vi "Fetch Waveform Measurement.vi"(6 "Source 2 (21: None)":u16(ring)=21 items=["Channel 1", "Channel 2", "Channel 3", "Channel 4", "DIG 0", "DIG 1", "DIG 2", "DIG 3", "DIG 4", "DIG 5", "DIG 6", "DIG 7", "DIG 8", "DIG 9", "DIG 10", "DIG 11", "DIG 12", "DIG 13", "DIG 14", "DIG 15", "Math", "None"], 8 "error in (no error)":errorcluster, 9 "Measurement Function (7: Frequency)":u16(ring)=7 items=["Amplitude", "Voltage Average", "Base", "Counter", "Delay", "Duty Cycle", "Fall Time", "Frequency", "Voltage Max", "Voltage Min", "Overshoot", "Voltage Vpp", "Period", "Phase", "Preshoot", "Rise Time", "Voltage RMS", "Top", "Width Positive", "X at Max Y", "X at Min Y"], 10 "Source 1 (0: Channel 1)":u16(ring) items=["Channel 1", "Channel 2", "Channel 3", "Channel 4", "DIG 0", "DIG 1", "DIG 2", "DIG 3", "DIG 4", "DIG 5", "DIG 6", "DIG 7", "DIG 8", "DIG 9", "DIG 10", "DIG 11", "DIG 12", "DIG 13", "DIG 14", "DIG 15", "Math"], 11 "VISA resource name":refnum<visa-resource-name>) -> (0 "error out":errorcluster, 2 "Measured Value":dbl, 3 "VISA resource name out":refnum<visa-resource-name>)   [LabVIEW 2018, in "Agilent 6000 Series.lvlib"]
doc: "This VI obtains a waveform measurement and returns the measurement value. You specify a particular measurement type, such as rise time, frequency, and voltage peak-to-peak. The waveform on which the oscilloscope calculates the waveform measurement is from an acquisition that you previously initiated. \n\nUse the ag6000 Initiate Acquisition.vi to start an acquisition on the channels that you enable with the ag6000 Configure Channel.vi. The oscilloscope acquires waveforms for the enabled channels concurrently. You use the ag6000 Acquisition Status.vi to determine when the acquisition is complete. You call this VI separately for each waveform measurement you want to obtain on a specific channel.\n\nYou can call the ag6000 Read Waveform Measurement.vi instead of the ag6000 Initiate Acquisition.vi. The ag6000 Read Waveform Measurement.vi starts an acquisition on all enabled channels. It then waits for the acquisition to complete, obtains a waveform measurement on the channel you specify, and returns the measurement value. You call this VI separately for any other waveform measurement that you want to obtain on a specific channel.\n\nNotes:\n\n(1) You must configure the appropriate reference levels before you call this VI to take a rise time, fall time, width negative, width positive, duty cycle negative, or duty cycle positive measurement.\n\n(2) You configure the low, mid, and high references either by calling the ag6000 Configure Reference Levels.vi.\n\n\n(3) This VI does not check the instrument status. Typically, you call this VI only in a sequence of calls to other low-level driver VIs. The sequence performs one operation. You use the low-level VIs to optimize one or more aspects of interaction with the instrument. If you want to check the instrument status, call the ag6000 Error-Query.vi at the conclusion of the sequence."
uses:
  Agilent 6000 Series.lvlib
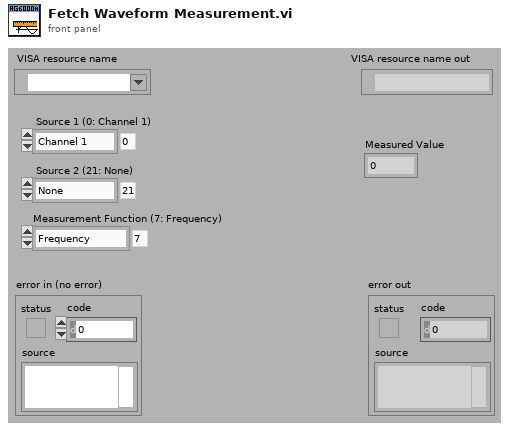
[diagram p1: front panel]
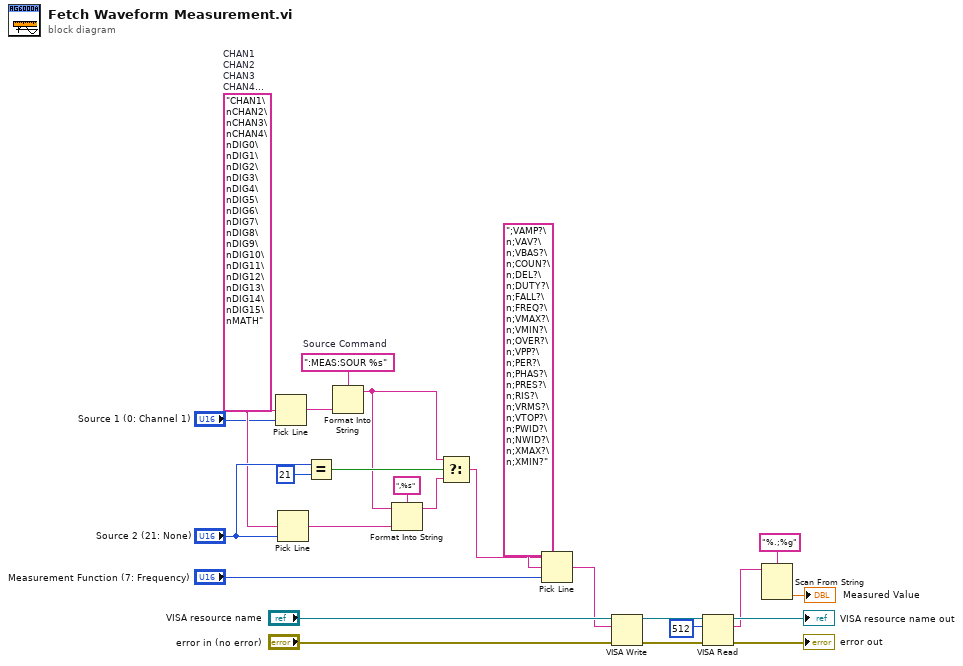
[diagram p0: block diagram]
diagram:
  w13 = ":MEAS:SOUR %s"  # Source Command
  w4 = "CHAN1\nCHAN2\nCHAN3\nCHAN4\nDIG0\nDIG1\nDIG2\nDIG3\nDIG4\nDIG5\nDIG6\nDIG7\nDIG8\nDIG9\nDIG10\nDIG11\nDIG12\nDIG13\nDIG14\nDIG15\nMATH"  # CHAN1 CHAN2 CHAN3 CHAN4 DIG0 DIG1 DIG2 DIG3 DIG4 DIG5 DIG6 DIG7 DIG8 DIG9 DIG10 DIG11 DIG12 DIG13 DIG14 DIG15 MATH
  n1 = Pick Line(multi-line string=w4, line index="Source 1 (0: Channel 1)") -> (output string=w12:string)  [unwired: 1 in]
  n2 = Pick Line(multi-line string=w4, line index="Source 2 (21: None)") -> (output string=w7:string)  [unwired: 1 in]
  n3 = Equal?(x="Source 2 (21: None)", y=u16 21) -> (x = y?=w11:bool)
  n4 = Format Into String(format string=w13, w12) -> (resulting string=w5:string)  [unwired: 2 in, 1 out]
  n5 = Format Into String(format string=",%s", initial string=w5, w7) -> (resulting string=w6:string)  [unwired: 1 in, 1 out]
  n6 = Select(t=w5, s=w11, f=w6) -> (s? t:f=w1:string)
  n7 = Pick Line(string ("")=w1, multi-line string=";VAMP?\n;VAV?\n;VBAS?\n;COUN?\n;DEL?\n;DUTY?\n;FALL?\n;FREQ?\n;VMAX?\n;VMIN?\n;OVER?\n;VPP?\n;PER?\n;PHAS?\n;PRES?\n;RIS?\n;VRMS?\n;VTOP?\n;PWID?\n;NWID?\n;XMAX?\n;XMIN?", line index="Measurement Function (7: Frequency)") -> (output string=w2:string)
  n8 = VISA Write(VISA resource name="VISA resource name", write buffer=w2, error in (no error)="error in (no error)") -> (VISA resource name out=w20:refnum<visa-resource-name>, error out=w21:errorcluster)  [unwired: 1 out]
  n9 = VISA Read(VISA resource name=w20, byte count=u32 512, error in (no error)=w21) -> (VISA resource name out=→"VISA resource name out":refnum<visa-resource-name>, read buffer=w15:string, error out=→"error out":errorcluster)  [unwired: 1 out]
  n10 = Scan From String(format string="%.;%g", input string=w15) -> (output 1=→"Measured Value":dbl)  [unwired: 3 in, 3 out]
